vi "Pair.vi"(8 "error in (no error)":errorcluster, 11 "BT in":refnum<class "BT.lvclass">) -> (0 "error out":errorcluster, 3 "BT out":refnum<class "BT.lvclass">)   [LabVIEW 2014, in "BT.lvlib" / "BT.lvclass"]
uses:
  BT.lvclass
  BT.lvclass/BT.ctl
  C:/Users/yang/Desktop/BT Connect/InTheHand.Net.Personal.dll
  BT Connect/InTheHand.Net.Personal.dll
panel:
  in  "Pin":string
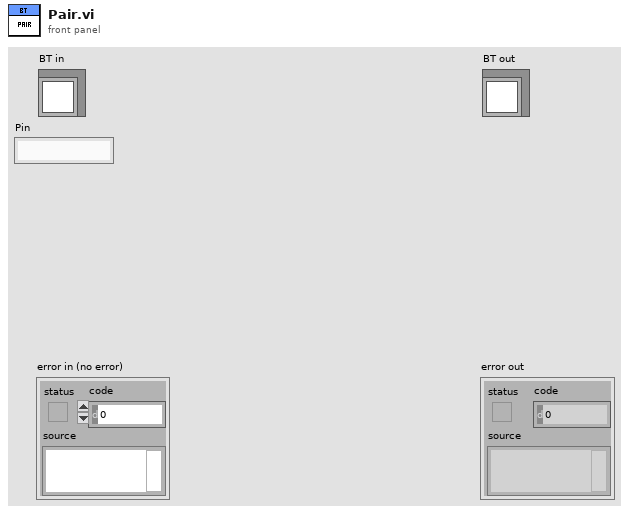
[diagram p1: front panel]
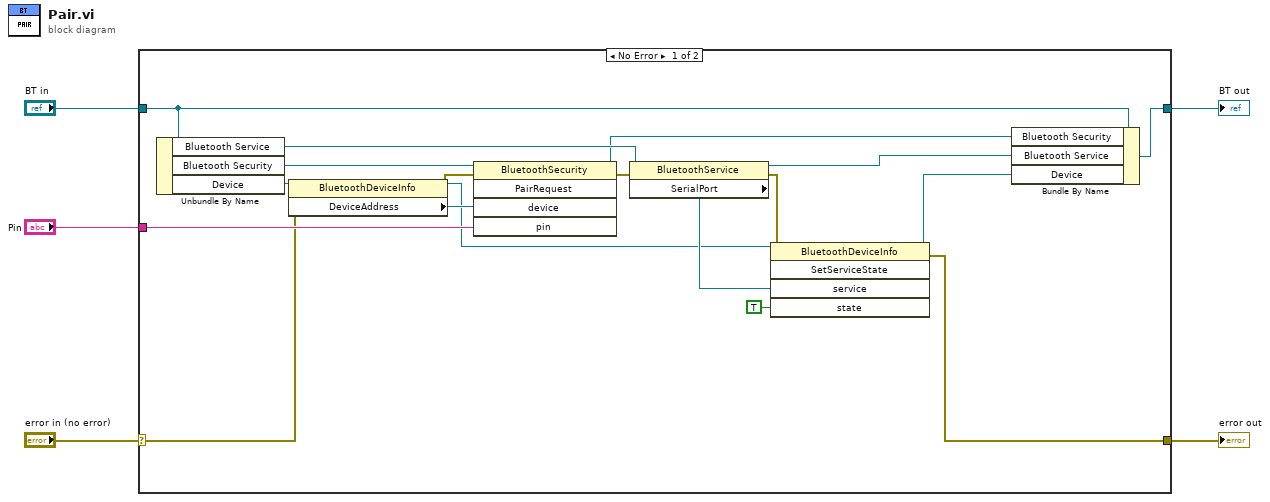
[diagram p0: block diagram]
diagram:
  n1 = case shown="No Error" "error in (no error)" {
    selector: "error in (no error)" -> [w16 w25]
    tunnel: [w11 w25] -> w4
    tunnel: [w7 w24] -> w2
    tunnel: "BT in" -> [w8 w24]
    tunnel: "Pin" -> [w20 _]
    frame No Error {
      n2 = Unbundle By Name(w8) -> ("Bluetooth Service"=w19:refnum<k24>, "Bluetooth Security"=w23:refnum<k24>, "Device"=w22:refnum<k24>)
      n3 = property class="BluetoothDeviceInfo"(reference=w22, error in=w16) -> (reference out=w13:refnum<k24>, error out=w17:errorcluster, "DeviceAddress"=w21:refnum<k24>)
      n4 = invoke class="BluetoothSecurity" method="PairRequest"(reference=w23, error in=w17, "device"=w21, "pin"=w20) -> (reference out=w10:refnum<k24>, error out=w18:errorcluster)  [unwired: 1 in, 3 out]
      n5 = property class="BluetoothService"(reference=w19, error in=w18) -> (reference out=w9:refnum<k24>, error out=w15:errorcluster, "SerialPort"=w14:refnum<k24>)
      n6 = invoke class="BluetoothDeviceInfo" method="SetServiceState"(reference=w13, error in=w15, "service"=w14, "state"=TRUE) -> (reference out=w6:refnum<k24>, error out=w11:errorcluster)  [unwired: 1 in, 3 out]
      n7 = Bundle By Name(cluster=w8, "Bluetooth Security"=w10, "Bluetooth Service"=w9, "Device"=w6) -> (w7:refnum<class "BT.lvclass">)
    }
    frame Error {
    }
  }
  "error out" <- w4
  "BT out" <- w2
